vi "File to Array.vi"(8 "error in":errorcluster, 11 "file path in":path) -> (0 "error out":errorcluster, 2 "list out":T1[](array[typedef]) {"Creation Date" format="%<%x>T"; "Last Updated" format="%<%x>T"}, 3 "file path out":path)   [LabVIEW 2018]
uses:
  Type Defs/SR Cluster.ctl
  Type Defs/SR Status.ctl
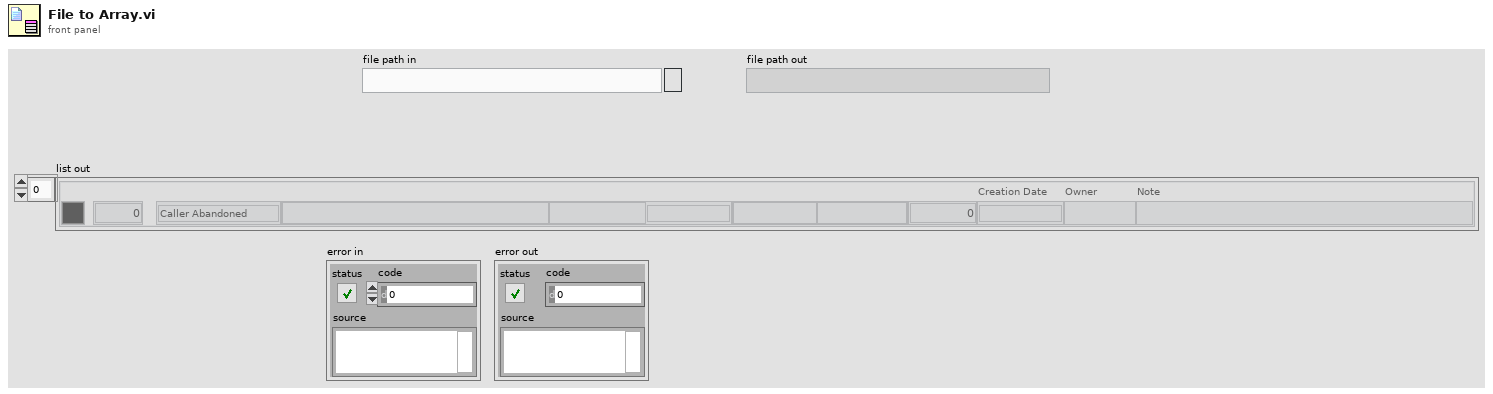
[diagram p1: front panel]
types:
  T1 = typedef "SR Cluster.ctl" = cluster{"Color":u32, "SR Number":i32, "SR Status":T2, "Name":string, "Summary":string, "Last Updated":timestamp, "SR Type":string, "Service Level":string, "Days Open":dbl, "Creation Date":timestamp, "Owner":string, "Note":string}
  T2 = typedef "SR Status.ctl" = enum16{"Caller Abandoned", "Created in Error", "Expired", "Forum Resolved AE", "Forum Resolved Customer", "IN WORK", "IN WORK Collab with AES", "IN WORK Collab with PSE", "IN WORK Collab with SE", "IN WORK Customer Added Note", "IN WORK Escalation", "IN WORK Wait on Customer", "Open", "Potentially Resolved", "Presumed Resolved", "RMA Approved for Return", "RMA Closed", "RMA Closed - DOA", "RMA In Progress", "RMA Open", "RMA Waiting on Customer", "Resolved", "Passed Off"}
  T3 = enum16{"open", "replace", "create", "open or create", "replace or create", "replace or create with confirmation"}
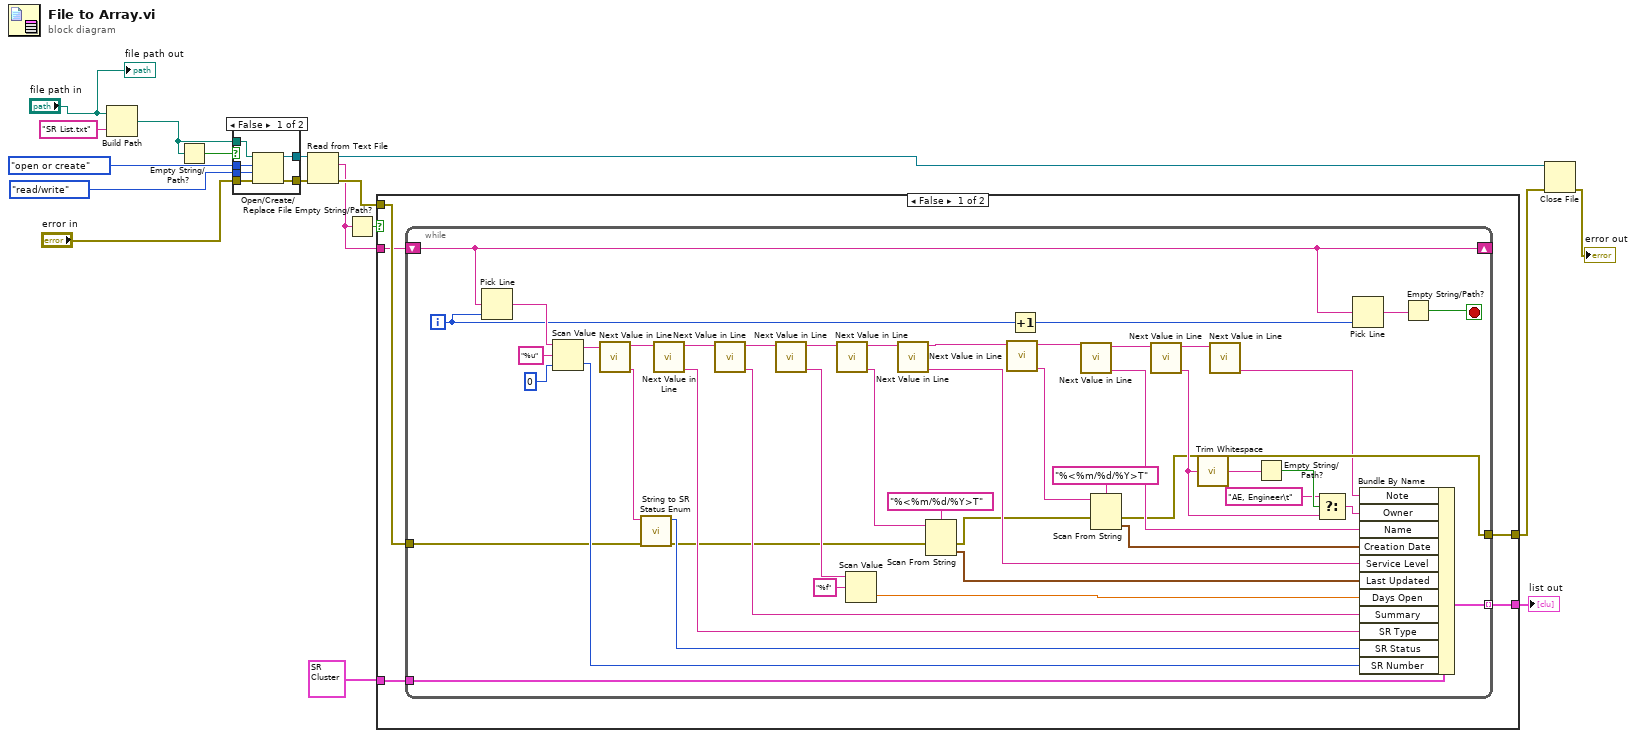
[diagram p0: block diagram]
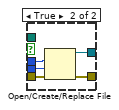
[diagram p2: hidden frame]
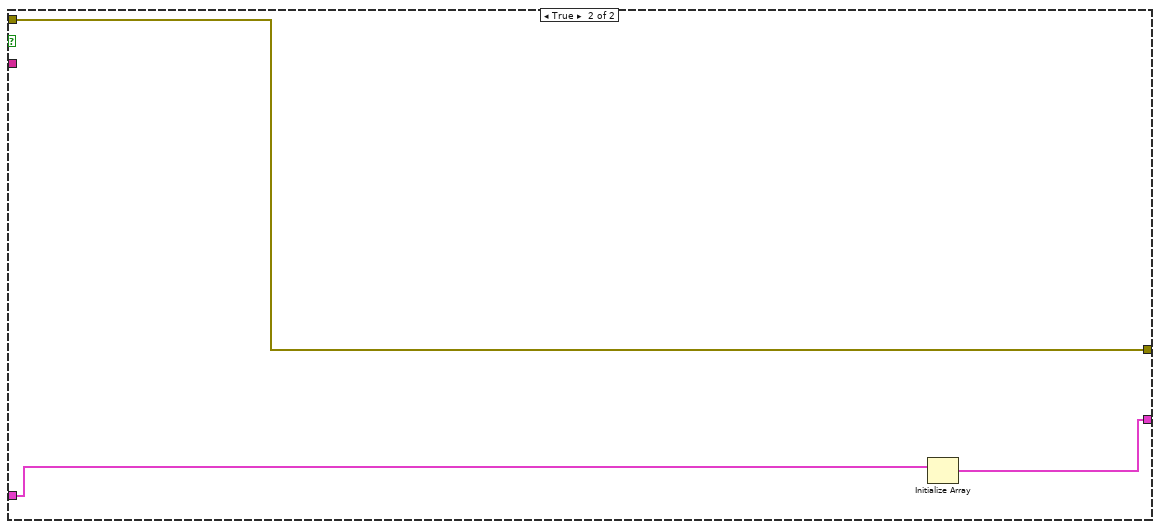
[diagram p3: hidden frame]
diagram:
  n1 = Build Path(base path="file path in", name or relative path="SR List.txt") -> (appended path=w2:path)
  n2 = Empty String/Path?(string/path=w2) -> (empty?=w4:bool)
  n3 = case shown="False" w4 {
    tunnel: enum16{"read/write", "read-only", "write-only"}."read/write" ("access (0:read/write)") -> [w23 w27]
    tunnel: T3."open or create" ("operation (0:open)") -> [w22 w28]
    tunnel: "error in" -> [w21 w26]
    tunnel: [w20 w24] -> w14
    tunnel: [w19 w25] -> w13
    tunnel: w2 -> [w18 _]
    frame False {
      n4 = Open/Create/Replace File(file path (use dialog)=w18, error in=w21, operation (0:open)=w22, access (0:read/write)=w23) -> (refnum out=w20:refnum<file>, error out=w19:errorcluster)  [unwired: 2 in, 1 out]
    }
    frame True {
      n5 = Open/Create/Replace File(error in=w26, operation (0:open)=w28, access (0:read/write)=w27) -> (refnum out=w24:refnum<file>, error out=w25:errorcluster)  [unwired: 3 in, 1 out]
    }
  }
  n6 = Read from Text File(file (use dialog)=w14, error in=w13) -> (refnum out=w8:refnum<file>, text=w10:string, error out=w11:errorcluster)  [unwired: 2 in, 1 out]
  n7 = Empty String/Path?(string/path=w10) -> (empty?=w12:bool)
  n8 = case shown="False" w12 {
    tunnel: w11 -> [w32 w80]
    tunnel: w10 -> [w31 _]
    tunnel: T1 {"Color"=0, "SR Number"=0, "SR Status"=enum."Caller Abandoned", "Name"="", "Summary"="", "Last Updated"=timestamp(0 s since 1904-01-01), "SR Type"="", "Service Level"="", "Days Open"=0.0, "Creation Date"=timestamp(0 s since 1904-01-01), "Owner"="", "Note"=""} ("SR Cluster") -> [w33 w82]
    tunnel: [w30 w80] -> w7
    tunnel: [w29 w81] -> w6
    frame False {
      n9 = while {
        tunnel: w33 -> [w70]
        tunnel: w32 -> [w51]
        shift-right: [w58] -> _
        shift-left: w31 -> [w58]
        tunnel: [w59] -> w29 mode=indexing
        tunnel: [w36] -> w30
        i -> [w55]
        stop <- w56 stop-if-true
        n10 = Pick Line(multi-line string=w58, line index=w55) -> (output string=w79:string)  [unwired: 1 in]
        n11 = Scan Value(string=w79, format string="%u", default (0 dbl)=0) -> (output string=w76:string, value=w69:i32)
        n12 = call "Next Value in Line.vi"("string in"=w76) -> ("value"=w53:string, "rest of string"=w75:string)  [unwired: 9 in]
        n13 = call "String to SR Status Enum.vi"("error in"=w51, "string in"=w53) -> ("error out"=w50:errorcluster, "SR Status"=w52:T2)  [unwired: 8 in]
        n14 = call "Next Value in Line.vi"("string in"=w75) -> ("value"=w68:string, "rest of string"=w74:string)  [unwired: 9 in]
        n15 = call "Next Value in Line.vi"("string in"=w74) -> ("value"=w67:string, "rest of string"=w73:string)  [unwired: 9 in]
        n16 = call "Next Value in Line.vi"("string in"=w73) -> ("value"=w65:string, "rest of string"=w72:string)  [unwired: 9 in]
        n17 = call "Next Value in Line.vi"("string in"=w72) -> ("value"=w63:string, "rest of string"=w71:string)  [unwired: 9 in]
        n18 = Scan Value(string=w65, format string="%f") -> (value=w66:dbl)  [unwired: 1 in, 1 out]
        n19 = call "Next Value in Line.vi"("string in"=w71) -> ("value"=w60:string, "rest of string"=w49:string)  [unwired: 9 in]
        n20 = Scan From String(format string="%<%m/%d/%Y>T", input string=w63, error in=w50) -> (error out=w45:errorcluster, output 1=w61:timestamp)  [unwired: 2 in, 2 out]
        n21 = call "Next Value in Line.vi"("string in"=w49) -> ("value"=w48:string, "rest of string"=w44:string)  [unwired: 9 in]
        n22 = Increment(x=w55) -> (x+1=w54:i32)
        n23 = call "Next Value in Line.vi"("string in"=w44) -> ("value"=w43:string, "rest of string"=w42:string)  [unwired: 9 in]
        n24 = Scan From String(format string="%<%m/%d/%Y>T", input string=w48, error in=w45) -> (error out=w36:errorcluster, output 1=w46:timestamp)  [unwired: 2 in, 2 out]
        n25 = call "Next Value in Line.vi"("string in"=w42) -> ("value"=w37:string, "rest of string"=w35:string)  [unwired: 9 in]
        n26 = call <vilib>:"Trim Whitespace.vi"("string"=w37) -> ("trimmed string"=w41:string)  [unwired: 1 in]
        n27 = call "Next Value in Line.vi"("string in"=w35) -> ("value"=w34:string)  [unwired: 9 in, 1 out]
        n28 = Empty String/Path?(string/path=w41) -> (empty?=w40:bool)
        n29 = Select(t="AE, Engineer\t", s=w40, f=w37) -> (s? t:f=w38:string)
        n30 = Pick Line(multi-line string=w58, line index=w54) -> (output string=w57:string)  [unwired: 1 in]
        n31 = Bundle By Name(cluster=w70, "Note"=w34, "Owner"=w38, "Name"=w43, "Creation Date"=w46, "Service Level"=w60, "Last Updated"=w61, "Days Open"=w66, "Summary"=w67, "SR Type"=w68, "SR Status"=w52, "SR Number"=w69) -> (w59:T1)
        n32 = Empty String/Path?(string/path=w57) -> (empty?=w56:bool)
      }
    }
    frame True {
      n33 = Initialize Array(w82) -> (w81:T1[])  [unwired: 1 in]
    }
  }
  "list out" <- w6
  n34 = Close File(refnum=w8, error in=w7) -> (error out=→"error out":errorcluster)  [unwired: 1 out]
  "file path out" <- "file path in"
